vi "Delete Item.vi"(8 "错误输入":errorcluster, 9 "Mode":enum16{"End", "Begin"}(ring), 11 "Mlistbox Ref":refnum<vi>) -> (0 "错误输出":errorcluster, 3 "Mlistbox Ref Dup":refnum<vi>)   [LabVIEW 2012, in "Mlistbox Tools.lvlib"]
uses:
  Mlistbox Tools.lvlib
  ListBox/Custom Type/Read and Write Mode.ctl
  Property/Set and Get ItemNames.vi
  ListBox/Listbox Tool.lvlib
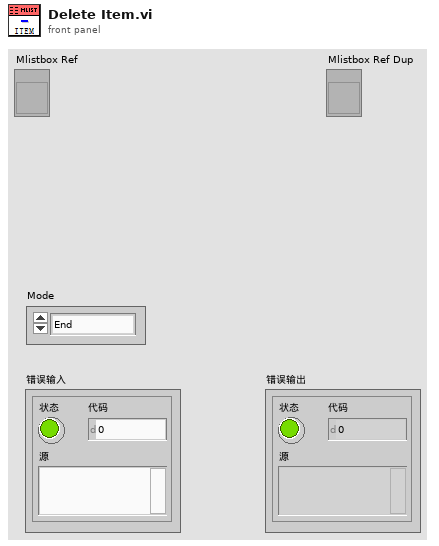
[diagram p1: front panel]
types:
  T1 = typedef "Listbox Tool.lvlib/Read and Write Mode.ctl" = enum16{"Read", "Write"}
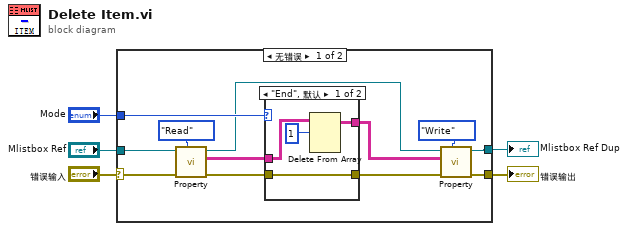
[diagram p0: block diagram]
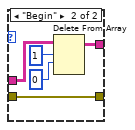
[diagram p2: hidden frame]
diagram:
  n1 = case shown="无错误" "错误输入" {
    selector: "错误输入" -> [w11 w28]
    tunnel: [w9 w28] -> w4
    tunnel: "Mlistbox Ref" -> [w17 w27]
    tunnel: "Mode" -> [w15 _]
    tunnel: [w10 w27] -> w1
    frame No Error {
      n2 = call-poly "Property.vi"("Mode"=Read_and_Write_Mode."Read", "错误输入"=w11, "Mlistbox Ref"=w17) -> ("错误输出"=w8:errorcluster, "ItemNames Out"=w14:string[][], "Mlistbox Ref Dup"=w6:refnum<vi>)  [unwired: 6 in]
      n3 = case shown="\"End\", 默认" w15 {
        tunnel: w14 -> [w21 w24]
        tunnel: [w18 w22] -> w12
        tunnel: w8 -> [w20 w26]
        tunnel: [w20 w26] -> w7
        frame "End", Default {
          n4 = Delete From Array(array=w21, length=1 ("长度")) -> (array with subset deleted=w18:string[][])  [unwired: 2 in, 1 out]
        }
        frame "Begin" {
          n5 = Delete From Array(array=w24, length=1 ("长度"), index (row)=0 ("索引")) -> (array with subset deleted=w22:string[][])  [unwired: 1 in, 1 out]
        }
      }
      n6 = call-poly "Property.vi"("Mode"=Read_and_Write_Mode."Write", "错误输入"=w7, "ItemNames In"=w12, "Mlistbox Ref"=w6) -> ("错误输出"=w9:errorcluster, "Mlistbox Ref Dup"=w10:refnum<vi>)  [unwired: 5 in, 1 out]
    }
    frame Error {
    }
  }
  "Mlistbox Ref Dup" <- w1
  "错误输出" <- w4
